vi "daq_example_ai_dis_synch.vi"() -> ()   [LabVIEW 2015]
uses:
  <vilib>/DAQmx/read.llb/DAQmx Read (Digital 1D U32 1Chan NSamp).vi
  <vilib>/DAQmx/read.llb/DAQmx Read (Analog 1D Wfm NChan NSamp).vi
  <vilib>/DAQmx/create/channels.llb/DAQmx Create Channel (AI-Voltage-Basic).vi
  <vilib>/DAQmx/create/channels.llb/DAQmx Create Channel (DI-Digital Input).vi
  <vilib>/DAQmx/configure/timing.llb/DAQmx Timing (Sample Clock).vi
  <vilib>/DAQmx/miscellaneous.llb/DAQmx Fill In Error Info.vi
  <resource>/objmgr/daqmx.rc
panel:
  out "DI":u32[](graph) caption="Analog Inputs"
  out "AI":waveform(dbl)[](graph) caption="Analog Inputs"
  out "error out AI":errorcluster
  out "error out DI":errorcluster
  out "N Loops":i32
  in  "stop":bool
  out "Actual Sample Rate":dbl=1000.0 format="%0.2f"
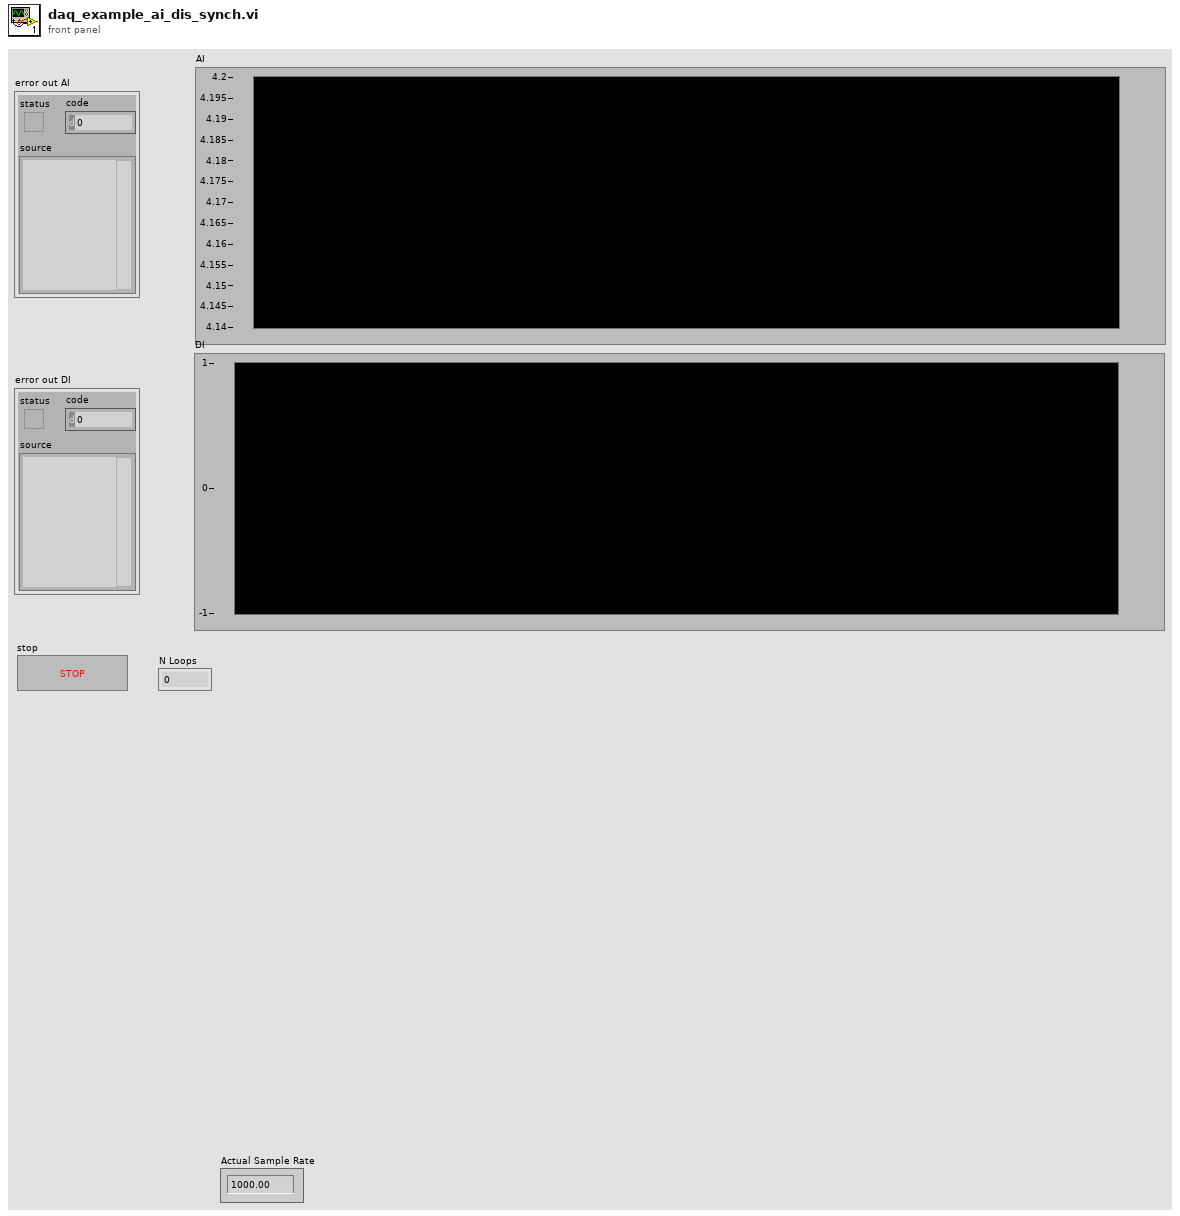
[diagram p1: front panel]
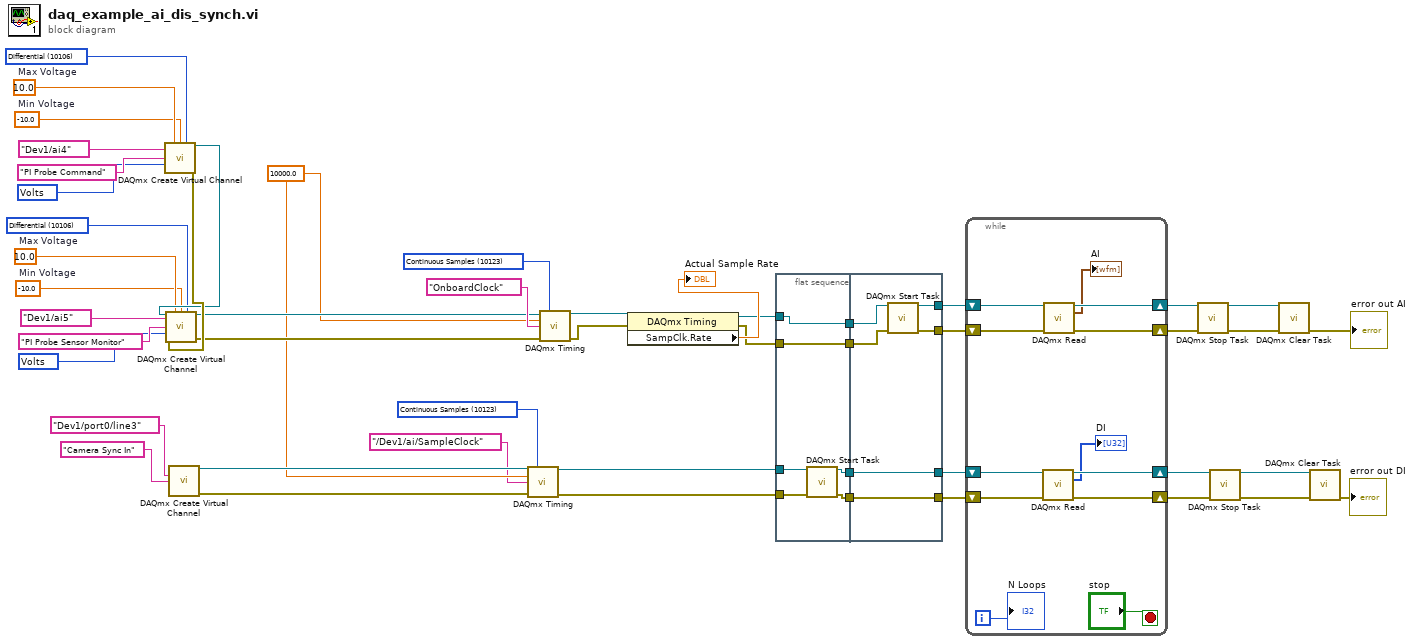
[diagram p0: block diagram]
diagram:
  w24 = 10000.0 ("Sample Rate")
  w27 = 10123 items=["Finite Samples"=10178, "Continuous Samples"=10123, "Hardware Timed Single Point"=12522] ("sample mode")
  w34 = 10123 items=["Finite Samples"=10178, "Continuous Samples"=10123] ("sample mode")
  w47 = 10348 items=["Volts"=10348, "From Custom Scale"=10065] ("units")
  w46 = 10106 items=["default"=-1, "RSE"=10083, "NRSE"=10078, "Differential"=10106, "Pseudodifferential"=12529] ("input terminal configuration")
  w44 = -10.0  # Min Voltage
  w45 = 10.0  # Max Voltage
  w42 = 10348 items=["Volts"=10348, "From Custom Scale"=10065] ("units")
  w41 = 10106 items=["default"=-1, "RSE"=10083, "NRSE"=10078, "Differential"=10106, "Pseudodifferential"=12529] ("input terminal configuration")
  w39 = -10.0  # Min Voltage
  w40 = 10.0  # Max Voltage
  n1 = call-poly <vilib>:"DAQmx Create Virtual Channel.vi"("maximum value"=w40, "minimum value"=w39, "input terminal configuration"=w41, "physical channels"=tag "Dev1/ai4", "name to assign"="PI Probe Command", "units"=w42) -> ("task out"=w49:refnum<k21>, "error out"=w50:errorcluster)  [unwired: 8 in]
  n2 = call-poly <vilib>:"DAQmx Create Virtual Channel.vi"("task in"=w49, "maximum value"=w45, "minimum value"=w44, "input terminal configuration"=w46, "physical channels"=tag "Dev1/ai5", "name to assign"="PI Probe Sensor Monitor", "units"=w47, "error in"=w50) -> ("task out"=w29:refnum<k21>, "error out"=w28:errorcluster)  [unwired: 6 in]
  n3 = call-poly <vilib>:"DAQmx Create Virtual Channel.vi"("lines"=tag "Dev1/port0/line3", "name to assign"="Camera Sync In") -> ("task out"=w26:refnum<k21>, "error out"=w25:errorcluster)  [unwired: 12 in]
  n4 = call-poly <vilib>:"DAQmx Timing.vi"("task/channels in"=w26, "sample mode"=w27, "rate"=w24, "source"=tag "/Dev1/ai/SampleClock", "error in"=w25) -> ("task out"=w22:refnum<k21>, "error out"=w21:errorcluster)  [unwired: 9 in]
  n5 = call-poly <vilib>:"DAQmx Timing.vi"("task/channels in"=w29, "sample mode"=w34, "rate"=w24, "source"=tag "OnboardClock" ("Sample Clock Source"), "error in"=w28) -> ("task out"=w38:refnum<k21>, "error out"=w37:errorcluster)  [unwired: 9 in]
  n6 = property class="DAQmx Timing"(reference=w38, error in=w37) -> (reference out=w19:refnum<k21>, error out=w17:errorcluster, "SampClk.Rate"=→"Actual Sample Rate":dbl)
  n7 = flat-sequence {
    tunnel: w22 -> [w56]
    tunnel: w21 -> [w55]
    tunnel: [w54] -> w20
    tunnel: w19 -> [w54]
    tunnel: [w53] -> w18
    tunnel: w17 -> [w53]
    tunnel: [w52] -> w14
    tunnel: [w51] -> w11
    tunnel: w20 -> [w62]
    tunnel: w18 -> [w61]
    tunnel: [w60] -> w16
    tunnel: [w59] -> w15
    tunnel: w14 -> [w58]
    tunnel: [w58] -> w13
    tunnel: [w57] -> w12
    tunnel: w11 -> [w57]
    frame #0 {
      n8 = call <vilib>:"DAQmx Start Task.vi"("task/channels in"=w56, "error in"=w55) -> ("task out"=w52:refnum<k21>, "error out"=w51:errorcluster)  [unwired: 12 in]
    }
    frame #1 {
      n9 = call <vilib>:"DAQmx Start Task.vi"("task/channels in"=w62, "error in"=w61) -> ("task out"=w60:refnum<k21>, "error out"=w59:errorcluster)  [unwired: 12 in]
    }
  }
  n10 = while {
    shift-right: [w70] -> w10
    shift-left: w16 -> [w74]
    shift-right: [w69] -> w9
    shift-left: w15 -> [w73]
    shift-right: [w68] -> w8
    shift-left: w13 -> [w72]
    shift-right: [w67] -> w7
    shift-left: w12 -> [w71]
    i -> [w65]
    stop <- "stop" stop-if-true
    n11 = call-poly <vilib>:"DAQmx Read.vi"("task/channels in"=w72, "error in"=w71) -> ("task out"=w68:refnum<k21>, "data"=→"DI":u32[], "error out"=w67:errorcluster)  [unwired: 11 in]
    n12 = call-poly <vilib>:"DAQmx Read.vi"("task/channels in"=w74, "error in"=w73) -> ("task out"=w70:refnum<k21>, "data"=→"AI":waveform(dbl)[], "error out"=w69:errorcluster)  [unwired: 11 in]
    "N Loops" <- w65
  }
  n13 = call <vilib>:"DAQmx Stop Task.vi"("task/channels in"=w10, "error in"=w9) -> ("task out"=w6:refnum<k21>, "error out"=w5:errorcluster)  [unwired: 12 in]
  n14 = call <vilib>:"DAQmx Stop Task.vi"("task/channels in"=w8, "error in"=w7) -> ("task out"=w4:refnum<k21>, "error out"=w3:errorcluster)  [unwired: 12 in]
  n15 = call <vilib>:"DAQmx Clear Task.vi"("task in"=w6, "error in"=w5) -> ("error out"=→"error out AI":errorcluster)  [unwired: 13 in]
  n16 = call <vilib>:"DAQmx Clear Task.vi"("task in"=w4, "error in"=w3) -> ("error out"=→"error out DI":errorcluster)  [unwired: 13 in]
